vi "GetCalibrationResultList.vi"(8 "error in (no error)":errorcluster, 11 "ByteGSWebAPI-V0 in":refnum<class "ByteGSWebAPI-V0.lvclass">) -> (0 "error out":errorcluster, 2 "CalibrationResultsList":T1, 3 "ByteGSWebAPI-V0 out":refnum<class "ByteGSWebAPI-V0.lvclass">, 4 "body":string, 6 "headers":string)   [LabVIEW 2019, in "ByteGSWebAPI.lvlib" / "ByteGSWebAPI-V0.lvclass"]
uses:
  ByteGSWebAPI-V0.lvclass
  Cntrls/MultipleCalibrationResults.ctl
  Cntrls/SingleCalibrationResult.ctl
  54c15d21-1fd3-4ea8-80e2-c69b0da6434b.vi
  <vilib>/JDP Science/JSONtext/JSON text to Variant.vi
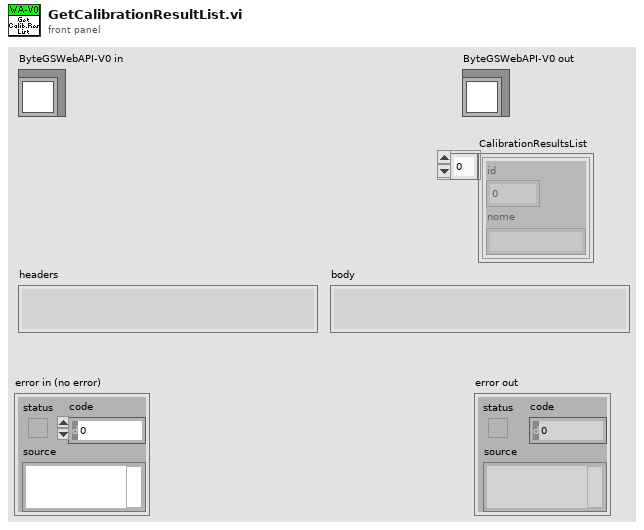
[diagram p1: front panel]
types:
  T1 = typedef "ByteGSWebAPI.lvlib/ByteGSWebAPI-V0.lvclass/MultipleCalibrationResults.ctl" = T2[]
  T2 = typedef "ByteGSWebAPI.lvlib/ByteGSWebAPI-V0.lvclass/SingleCalibrationResult.ctl" = cluster{"id":i32, "nome":string}
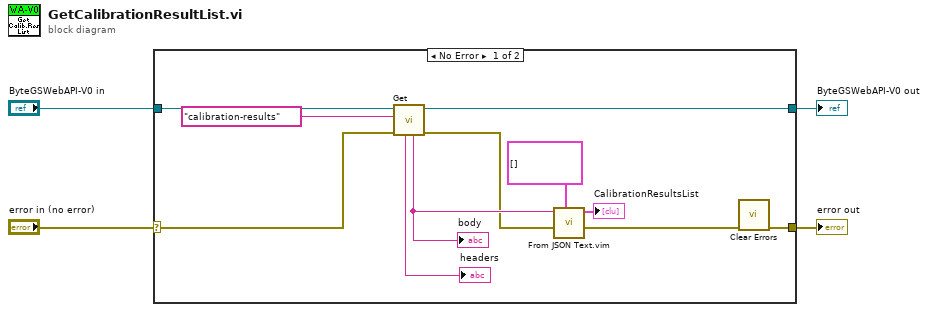
[diagram p0: block diagram]
diagram:
  n1 = case shown="No Error" "error in (no error)" {
    selector: "error in (no error)" -> [w12 w17]
    tunnel: [w7 w17] -> w3
    tunnel: [w14 w16] -> w1
    tunnel: "ByteGSWebAPI-V0 in" -> [w15 w16]
    frame No Error {
      n2 = call-dynamic "Get.vi"("error in (no error)"=w12, "Request"="calibration-results" ("Parameter"), "ByteGSWebAPI-V0 in"=w15) -> ("error out"=w9:errorcluster, "ByteGSWebAPI-V0 out"=w14:refnum<class "ByteGSWebAPI-V0.lvclass">, "body"=w10:string, "headers"=→"headers":string)  [unwired: 5 in]
      "body" <- w10
      n3 = call "From JSON Text.vim"("Data Type and Default Value"=T1 [] ("MultipleCalibrationResults"), "error in (no error)"=w9, "JSON"=w10) -> ("error out"=w8:errorcluster, "Data out"=→"CalibrationResultsList":T1)  [unwired: 7 in]
      n4 = call <vilib>:"Clear Errors.vi"("error in (no error)"=w8) -> ("error out"=w7:errorcluster)  [unwired: 5 in, 1 out]
    }
    frame Error {
    }
  }
  "error out" <- w3
  "ByteGSWebAPI-V0 out" <- w1
